vi "Order tree.vi"(7 "Tags map":refnum<vi>, 8 "error in":errorcluster, 11 "TreeControl in":refnum<vi>) -> (0 "error out":errorcluster)   [LabVIEW 2025, in "CAN-LIN Raw Bus Capture UI.lvlib"]
uses:
  CAN-LIN Raw Bus Capture UI.lvlib
  Table_Filtering/Table_Filtering.lvlib
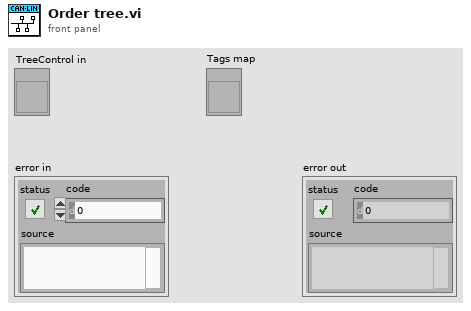
[diagram p1: front panel]
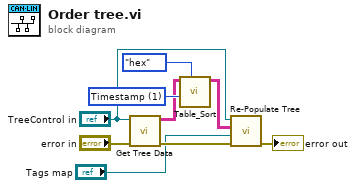
[diagram p0: block diagram]
diagram:
  w9 = u16 1 items=["Packet_Number", "Timestamp", "Source", "Destination", "Protocol", "Length", "Data"] ("Sort by")
  n1 = call "Get Tree Data.vi"("error in"="error in", "Tree ref"="TreeControl in") -> ("error out"=w6:errorcluster, "Array"=w2:string[][])  [unwired: 8 in]
  n2 = call "Table_Sort.vi"("Sort Type"=enum16{"numerical", "hex", "string"}."hex", "Sort by"=w9, "Unsorted Data"=w2) -> ("Sorted data"=w3:string[][])  [unwired: 8 in]
  n3 = call "Re-Populate Tree.vi"("error in"=w6, "Tags map"="Tags map", "Data in"=w3, "TreeControl in"="TreeControl in") -> ("error out"=→"error out":errorcluster)  [unwired: 7 in]
